vi "SubProperty To Color.vi"(11 "Value":string) -> (3 "Color":u32)   [LabVIEW 2019, in "LSS.lvlib"]
doc: "Convert the value for the color input to a numeric representation that can be used by LabVIEW to set front panel object color values. This value input can be either a hexidecimal representation of the number, or a string mnemonic that will be parsed out of the colorMap.\n\n<b>Inputs:</b>\n<b>Value</b> - The parsed value section of the LSS string. This is the data that will be converted by this VI.\n\n<b>Outputs:</b>\n<b>Color</b> - The numeric representation of the string passed in by value."
uses:
  LSS.lvlib
  Controls/Mode.ctl
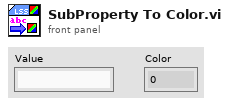
[diagram p1: front panel]
types:
  T1 = typedef "LSS.lvlib/Mode.ctl" = enum16{"Write", "Add", "Read"}
  T2 = typedef "LSS.lvlib/colorMap.ctl" = cluster{"color-name":string, "hex-value":string}
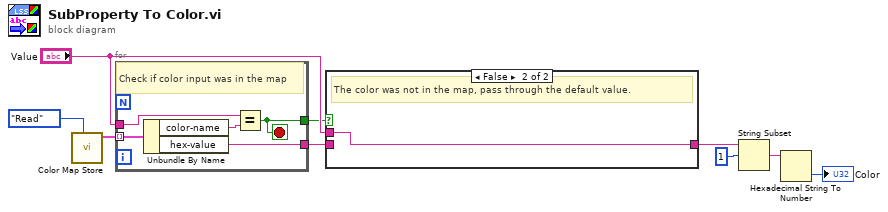
[diagram p0: block diagram]
diagram:
  n1 = call "Color Map Store.vi"("Mode"=Mode."Read") -> ("colorMap"=w9:T2[])  [unwired: 8 in, 2 out]
  n2 = for {
    tunnel: w9 -> [w14] mode=indexing
    tunnel: "Value" -> [w13]
    tunnel: [w11] -> w7
    tunnel: [w10] -> w4
    stop <- w10 stop-if-true
    # "Check if color input was in the map"
    n3 = Unbundle By Name(w14) -> ("color-name"=w12:string, "hex-value"=w11:string)
    n4 = Equal?(x=w13, y=w12) -> (x = y?=w10:bool)
  }
  n5 = case shown="False" w4 {
    tunnel: [w15 w16] -> w3
    tunnel: w7 -> [w15 _]
    tunnel: "Value" -> [_ w16]
    frame True {
      # "The color was in the map, use the switched value."
    }
    frame False {
      # "The color was not in the map, pass through the default value."
    }
  }
  n6 = String Subset(string=w3, offset (0)=1) -> (substring=w5:string)  [unwired: 1 in]
  n7 = Hexadecimal String To Number(string=w5) -> (number=→"Color":u32)  [unwired: 2 in, 1 out]
